vi "UpdateUserInterface.vi"(8 "error in (no error)":errorcluster, 10 "DataExchange":T1, 11 "DataLoggerUI in":refnum<class "DataLoggerUI.lvclass">) -> (0 "error out":errorcluster, 2 "DataExchange Out":T1, 3 "DataLoggerUI out":refnum<class "DataLoggerUI.lvclass">)   [LabVIEW 2020, in "DataLogger.lvlib" / "DataLoggerUI.lvlib" / "DataLoggerUI.lvclass"]
uses:
  DataLoggerUI.lvclass
  Hardware Abstraction Layer/Component/Device/Device/DataExchange.ctl
  DataLoggerUI.lvclass/DataLoggerUI.ctl
  <vilib>/vision/Image Controls.llb/IMAQ Image.ctl
  Hardware Abstraction Layer/Component/GenericActor/GenericActor/GenericController.lvclass
  Interface/DataListener/DataListener.lvclass
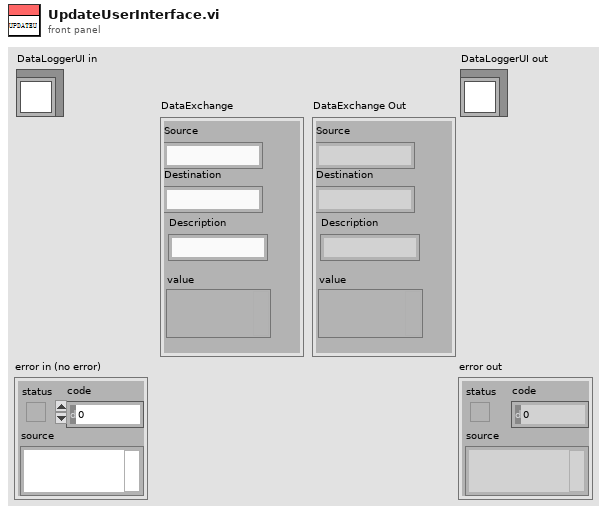
[diagram p1: front panel]
types:
  T1 = typedef "DataListener.lvclass/DataExchange.ctl" = cluster{"Source":string, "Destination":string, "Description":string, "value":variant}
  T2 = cluster{"StreamToDisk?":bool, "SingleStack?":bool, "Alert when finish?":bool, "TiffFileFullPath":path, "StreamFileFullPath":path}
  T3 = typedef "IMAQ Image.ctl" = refnum<image>
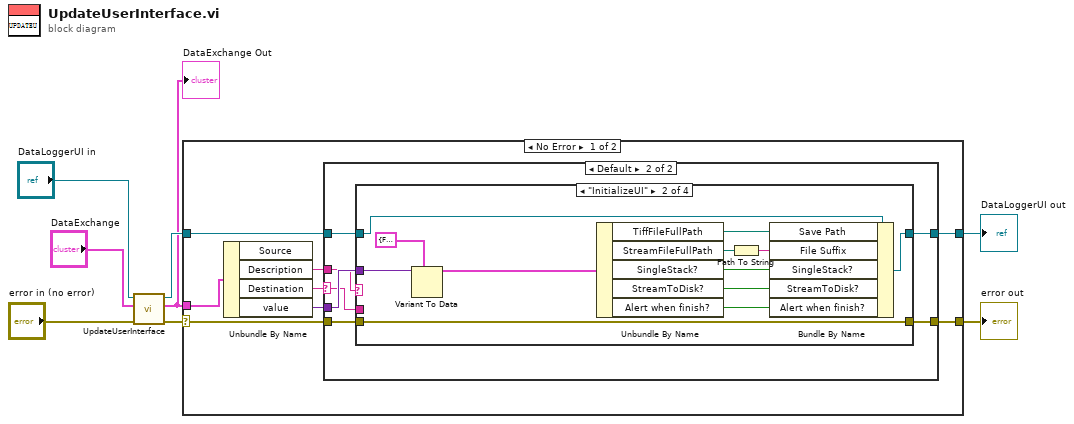
[diagram p0: block diagram]
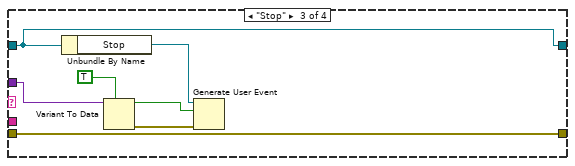
[diagram p4: hidden frame]
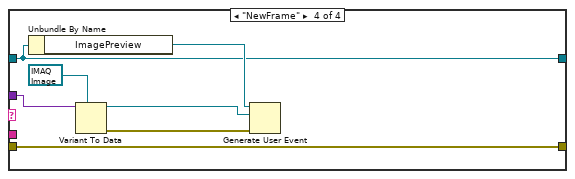
[diagram p5: hidden frame]
diagram:
  n1 = call-parent "UpdateUserInterface.vi"("error in (no error)"="error in (no error)", "DataExchange"="DataExchange", "GenericController in"="DataLoggerUI in") -> ("error out"=w4:errorcluster, "DataExchange Out"=w1:T1, "GenericController out"=w5:refnum<class "DataLoggerUI.lvclass">)  [unwired: 6 in]
  "DataExchange Out" <- w1
  n2 = case shown="No Error" w4 {
    selector: w4 -> [w11 w55]
    tunnel: [w10 w55] -> w2
    tunnel: [w12 w54] -> w3
    tunnel: w5 -> [w13 w54]
    tunnel: w1 -> [w16 _]
    frame No Error {
      n3 = Unbundle By Name(w16) -> ("Description"=w14:string, "Destination"=w9:string, "value"=w15:variant)  [unwired: 1 out]
      n4 = case shown="Default" w9 {
        selector: w9 -> [_ w19]
        tunnel: w15 -> [_ w25]
        tunnel: w14 -> [_ w24]
        tunnel: w13 -> [w18 w23]
        tunnel: [w18 w22] -> w12
        tunnel: w11 -> [w17 w21]
        tunnel: [w17 w20] -> w10
        frame "duplicate this case" {
        }
        frame Default {
          n5 = case shown="\"InitializeUI\"" w24 {
            tunnel: w25 -> [_ w37 w46 w53]
            tunnel: [w27 w36 w41 w50] -> w22
            tunnel: w23 -> [w27 w39 w41 w50]
            tunnel: [w26 w38 w40 w49] -> w20
            tunnel: w21 -> [w26 w38 w40 w49]
            tunnel: w19 -> [_ _ _ _]
            frame Default {
            }
            frame "InitializeUI" {
              n6 = Variant To Data(type=T2 {"StreamToDisk?"=FALSE, "SingleStack?"=FALSE, "Alert when finish?"=FALSE, "TiffFileFullPath"=path "", "StreamFileFullPath"=path ""} ("Images Saving"), Variant=w37) -> (data=w35:T2)  [unwired: 1 in, 1 out]
              n7 = Unbundle By Name(w35) -> ("TiffFileFullPath"=w30:path, "StreamFileFullPath"=w28:path, "SingleStack?"=w34:bool, "StreamToDisk?"=w33:bool, "Alert when finish?"=w32:bool)
              n8 = Path To String(path=w28) -> (string=w29:string)
              n9 = Bundle By Name(cluster=w39, "Save Path"=w30, "File Suffix"=w29, "SingleStack?"=w34, "StreamToDisk?"=w33, "Alert when finish?"=w32) -> (w36:refnum<class "DataLoggerUI.lvclass">)
            }
            frame "Stop" {
              n10 = Unbundle By Name(w41) -> ("Stop"=w45:refnum<user-event>)
              n11 = Variant To Data(type=TRUE, Variant=w46) -> (data=w44:bool, error out=w42:errorcluster)  [unwired: 1 in]
              n12 = Generate User Event(user event=w45, event data cluster=w44, error in=w42) -> ()  [unwired: 1 in, 2 out]
            }
            frame "NewFrame" {
              n13 = Unbundle By Name(w50) -> ("ImagePreview"=w52:refnum<user-event>)
              n14 = Variant To Data(type=T3 refnum ("event data"), Variant=w53) -> (data=w47:T3, error out=w51:errorcluster)  [unwired: 1 in]
              n15 = Generate User Event(user event=w52, event data cluster=w47, error in=w51) -> ()  [unwired: 1 in, 2 out]
            }
          }
        }
      }
    }
    frame Error {
    }
  }
  "error out" <- w2
  "DataLoggerUI out" <- w3
